vi "Create Transfer Group.vi"(4 "FIFO Options":T10, 5 "force inline? (F)":bool, 6 "Buffers":refnum<class "Buffers.lvclass">, 7 "id":i32, 8 "error in (no error)":errorcluster, 9 "Transfer Group Status":refnum<class "Status.lvclass">, 10 "Transfer Group configuration":T1={"name"="", "direction"=enum."Tx", "cycle timing"={"priority"=0, "decimation"=1, "offset"=0}, "thread index"=-1, "settings"=[], "Transfers"=[], "timeout behavior"=enum."Increment Late Count"} {"Transfers"."channels"."string offset" format="%d bytes"}, 11 "Transfers":refnum<class "Transfer.lvclass">[](array[class])) -> (0 "error out":errorcluster, 3 "Transfer Group out":refnum<class "Transfer Group.lvclass">)   [LabVIEW 2017, in "DSF Core.lvlib" / "Transfer Group.lvclass"]
uses:
  Transfer Group.lvclass
  Transfer/Transfer.lvclass
  Buffers/Buffers.lvclass
  Typedefs/DSF FIFO Options.ctl
  Typedefs/DSF Engine Transfer Group Configuration.ctl
  Typedefs/DSF Direction.ctl
  Typedefs/DSF Timing Info.ctl
  Typedefs/DSF Settings Info.ctl
  Typedefs/DSF Engine Transfer Configuration.ctl
  Typedefs/DSF Byte Order.ctl
  Typedefs/DSF Engine Channel Configuration.ctl
  Typedefs/DSF Data Type.ctl
  Typedefs/DSF Timeout Behavior.ctl
  Status/Status.lvclass
  Transfer Group.lvclass/Transfer Group.ctl
  Timing/Timing.lvclass
  DSF Core.lvlib
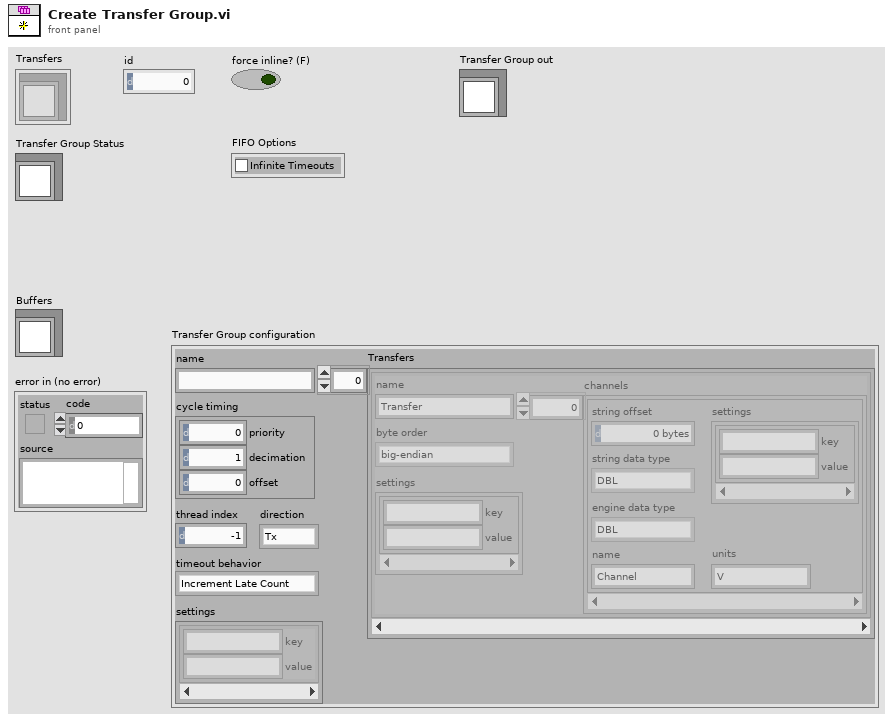
[diagram p1: front panel]
types:
  T1 = typedef "DSF Core.lvlib/DSF Engine Transfer Group Configuration.ctl" = cluster{"name":string, "direction":T2, "cycle timing":T3, "thread index":i32, "settings":T4, "Transfers":T5[], "timeout behavior":T9}
  T2 = typedef "DSF Core.lvlib/DSF Direction.ctl" = enum8{"Tx", "Rx"}
  T3 = typedef "DSF Core.lvlib/DSF Timing Info.ctl" = cluster{"priority":u64, "decimation":u64, "offset":u64}
  T4 = typedef "DSF Core.lvlib/DSF Settings Info.ctl" = cluster{"key":string, "value":string}[]
  T5 = typedef "DSF Core.lvlib/DSF Engine Transfer Configuration.ctl" = cluster{"name":string, "byte order":T6, "settings":T4, "channels":T7[]}
  T6 = typedef "DSF Core.lvlib/DSF Byte Order.ctl" = enum8{"big-endian", "little-endian"}
  T7 = typedef "DSF Core.lvlib/DSF Engine Channel Configuration.ctl" = cluster{"string offset":u64, "string data type":T8, "engine data type":T8, "name":string, "settings":T4, "units":string}
  T8 = typedef "DSF Core.lvlib/DSF Data Type.ctl" = enum8{"Bool", "SGL", "DBL", "I8", "I16", "I32", "I64", "U8", "U16", "U32", "U64"}
  T9 = typedef "DSF Core.lvlib/DSF Timeout Behavior.ctl" = enum8{"Increment Late Count", "Throw Error"}
  T10 = typedef "DSF Core.lvlib/DSF FIFO Options.ctl" = cluster{"Infinite Timeouts":bool}
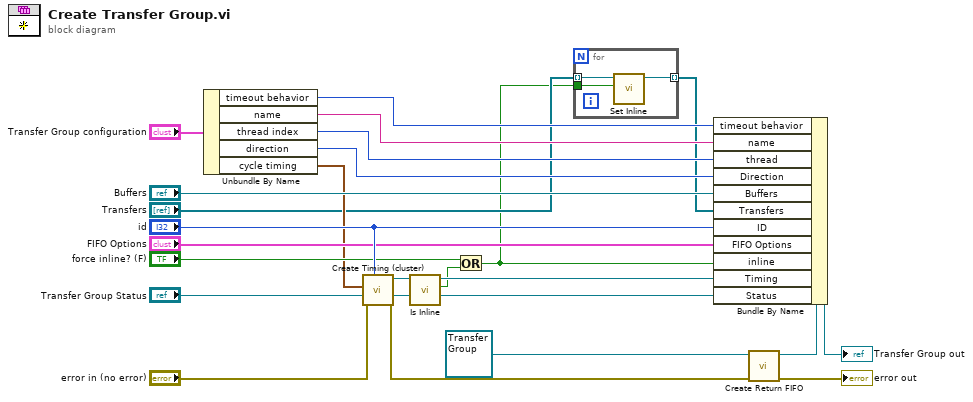
[diagram p0: block diagram]
diagram:
  n1 = Unbundle By Name("Transfer Group configuration") -> ("timeout behavior"=w5:T9, "name"=w6:string, "thread index"=w7:i32, "direction"=w8:T2, "cycle timing"=w9:T3)
  n2 = call "Create Timing (cluster).vi"("id (0)"="id", "error in (no error)"="error in (no error)", "cycle timing"=w9) -> ("error out"=w11:errorcluster, "Timing"=w16:refnum<class "Timing.lvclass">)  [unwired: 7 in]
  n3 = call "Is Inline.vi"("Timing in"=w16) -> ("inline?"=w14:bool, "Timing out"=w15:refnum<class "Timing.lvclass">)  [unwired: 9 in]
  n4 = Or(x="force inline? (F)", y=w14) -> (x .or. y?=w2:bool)
  n5 = for {
    tunnel: "Transfers" -> [w26] mode=indexing
    tunnel: w2 -> [w25]
    tunnel: [w24] -> w1 mode=indexing
    n6 = call "Set Inline.vi"("inline"=w25, "Transfer in"=w26) -> ("Transfer out"=w24:refnum<class "Transfer.lvclass">)  [unwired: 9 in]
  }
  n7 = call "Create Return FIFO.vi"("error in (no error)"=w11, "Transfer Group in"=refnum<class "Transfer Group.lvclass"> refnum ("Transfer Group type")) -> ("error out"=→"error out":errorcluster, "Transfer Group out"=w20:refnum<class "Transfer Group.lvclass">)  [unwired: 8 in]
  n8 = Bundle By Name(cluster=w20, "timeout behavior"=w5, "name"=w6, "thread"=w7, "Direction"=w8, "Buffers"="Buffers", "Transfers"=w1, "ID"="id", "FIFO Options"="FIFO Options", "inline"=w2, "Timing"=w15, "Status"="Transfer Group Status") -> (→"Transfer Group out":refnum<class "Transfer Group.lvclass">)
